vi "Configure.vi"(8 "error in (no error)":errorcluster, 11 "Template in":refnum<class "Template.lvclass">) -> (0 "error out":errorcluster, 2 "cancelled?":bool, 3 "Template out":refnum<class "Template.lvclass">)   [LabVIEW 2012, in "Template.lvclass"]
doc: "The configure method configures the details for the RabbitMQ connection. \n\nIn the derived class, make a call to the parent for setting these parameters."
uses:
  Template.lvclass
  Template.lvclass/Template.ctl
  <vilib>/Distrio/Murmex/Murmex/Murmex.lvclass
panel:
  in  "parameter":string
  in  "button:call parent":bool
  in  "button:ok":bool
  in  "button:cancel":bool
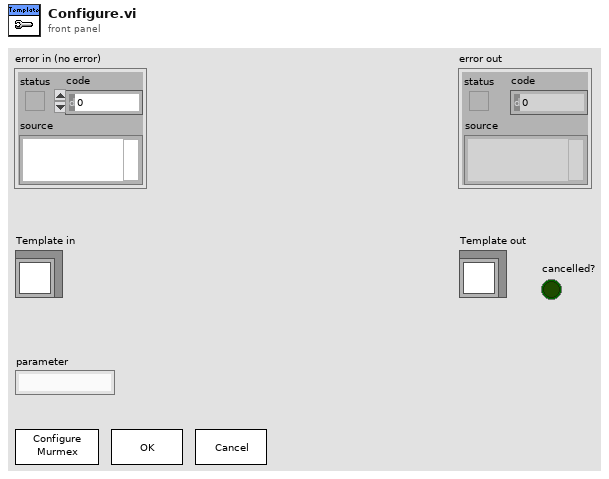
[diagram p1: front panel]
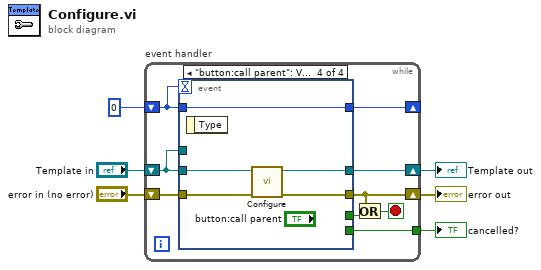
[diagram p0: block diagram]
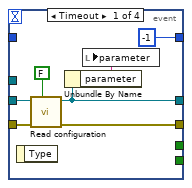
[diagram p2: hidden frame]
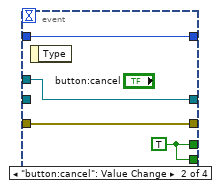
[diagram p3: hidden frame]
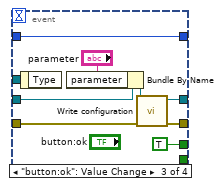
[diagram p4: hidden frame]
diagram:
  n1 = while "event handler" {
    tunnel: [w15] -> w5
    shift-right: [w14] -> w4
    shift-left: "Template in" -> [w12]
    shift-right: [w11] -> w6
    shift-left: "error in (no error)" -> [w13]
    shift-right: [w8] -> _
    shift-left: 0 -> [w7]
    stop <- w9 stop-if-true
    n2 = event shown="[3] \"button:call parent\": Value Change" {
      selector: _ -> [_ _ _ _]
      dyn-events: _ -> [_ _ _ _]
      timeout: w7 -> [_ _ _ _]
      tunnel: [w21 w25 w28 w37] -> w11
      tunnel: [_ w24 _ _] -> w15
      tunnel: [w18 w26 w30 w36] -> w14
      tunnel: w13 -> [w22 w25 w29 w38]
      tunnel: w12 -> [w20 _ w32 w39]
      tunnel: w12 -> [_ w26 _ _]
      tunnel: [_ w24 TRUE ("cancelled?") _] -> w10
      tunnel: [-1 w23 w27 w35] -> w8
      tunnel: w7 -> [_ w23 w27 w35]
      event Timeout {
        n3 = event-data() -> ()  [unwired: 1 in, 1 out]
        n4 = call-dynamic "Read configuration.vi"("force loading?"=FALSE, "error in (no error)"=w22, "Template in"=w20) -> ("error out"=w21:errorcluster, "Template out"=w18:refnum<class "Template.lvclass">)  [unwired: 7 in]
        n5 = Unbundle By Name(w18) -> ("parameter"=w17:string)
        n6 = local write "parameter"(w17) -> ()
      }
      event "button:cancel": Value Change {
        w24 = TRUE ("cancelled?")
        n7 = event-data() -> ()  [unwired: 1 in, 1 out]
      }
      event "button:ok": Value Change {
        n8 = event-data() -> ()  [unwired: 1 in, 1 out]
        n9 = Bundle By Name(cluster=w32, "parameter"="parameter") -> (w31:refnum<class "Template.lvclass">)
        n10 = call-dynamic "Write configuration.vi"("error in (no error)"=w29, "Template in"=w31) -> ("error out"=w28:errorcluster, "Template out"=w30:refnum<class "Template.lvclass">)  [unwired: 8 in]
      }
      event "button:call parent": Value Change {
        n11 = event-data() -> ()  [unwired: 1 in, 1 out]
        n12 = call-parent "Configure.vi"("error in (no error)"=w38, "Murmex in"=w39) -> ("error out"=w37:errorcluster, "Murmex out"=w36:refnum<class "Template.lvclass">)  [unwired: 7 in, 1 out]
      }
    }
    n13 = Or(x=w11, y=w10) -> (x .or. y?=w9:bool)
  }
  "error out" <- w6
  "Template out" <- w4
  "cancelled?" <- w5
